vi "TreeItem.Property.Set.vi"(4 "Set String as Binary":bool, 8 "error in (no error)":errorcluster, 9 "Value":variant, 10 "Property Name":string, 11 "BaseNodeType":refnum<k24>) -> (0 "error out":errorcluster, 1 "Replaced":bool, 3 "BaseNodeType":refnum<k24>)   [LabVIEW 2015, in "Advanced System Definition.lvlib"]
doc: "Saves the new values/items into their corresponding position within the Custom Device Hierarchy according to their corresponding data type."
uses:
  SysDef API/Advanced System Definition.lvlib
  NationalInstruments.VeriStand.SystemStorage
  _Types/Property.DependentFile.ctl
  <vilib>/NI Veristand/Custom Device API/Custom Device Item Ref.ctl
  NationalInstruments.VeriStand.SystemDefinitionAPI
  <vilib>/Utility/VariantDataType/VariantType.lvlib
  <vilib>/NI Veristand/Custom Device API/Custom Device API.lvlib
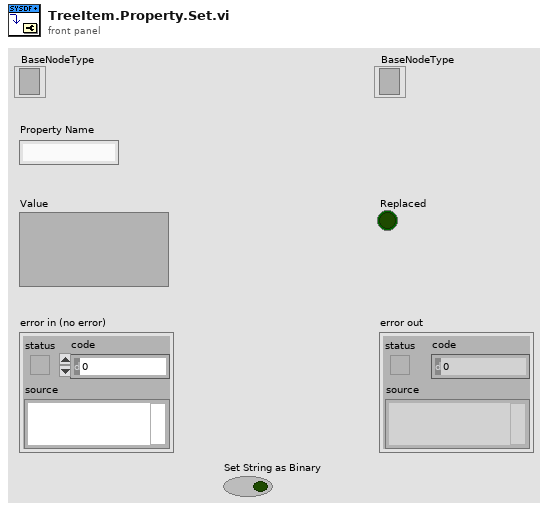
[diagram p1: front panel]
types:
  T1 = typedef "VariantType.lvlib/Type.ctl" = enum8{"Invalid Type", "Void", "I8", "I16", "I32", "I64", "U8", "U16", "U32", "U64", "Single Float", "Double Float", "Extended Float", "Single Complex", "Double Complex", "Extended Complex", "Enum U8", "Enum U16", "Enum U32", "Enum U64", "Single Float With Unit", "Double Float With Unit", "Extended Float With Unit", "Single Complex with Unit", "Double Complex with Unit", "Extended Complex with Unit", "Boolean", "String", "Path", "Picture", "Tag", "Array", "Cluster", "Variant", "LV Variant", "Waveform", "Timestamp", "Digital Waveform", "Digital Data", "ExpressData", "Refnum", "External Data", "VI", "Poly VI", "LabVIEW Class Instance", "Fixed Point"}
  T2 = typedef "Advanced System Definition.lvlib/Property.DependentFile.ctl" = cluster{"Original Path":path, "Version":string, "RTDestination":path, "ForceDownload":bool, "SupportedTarget":string, "MD5":string}
  T3 = typedef "Custom Device API.lvlib/Custom Device Item Ref.ctl" = u64
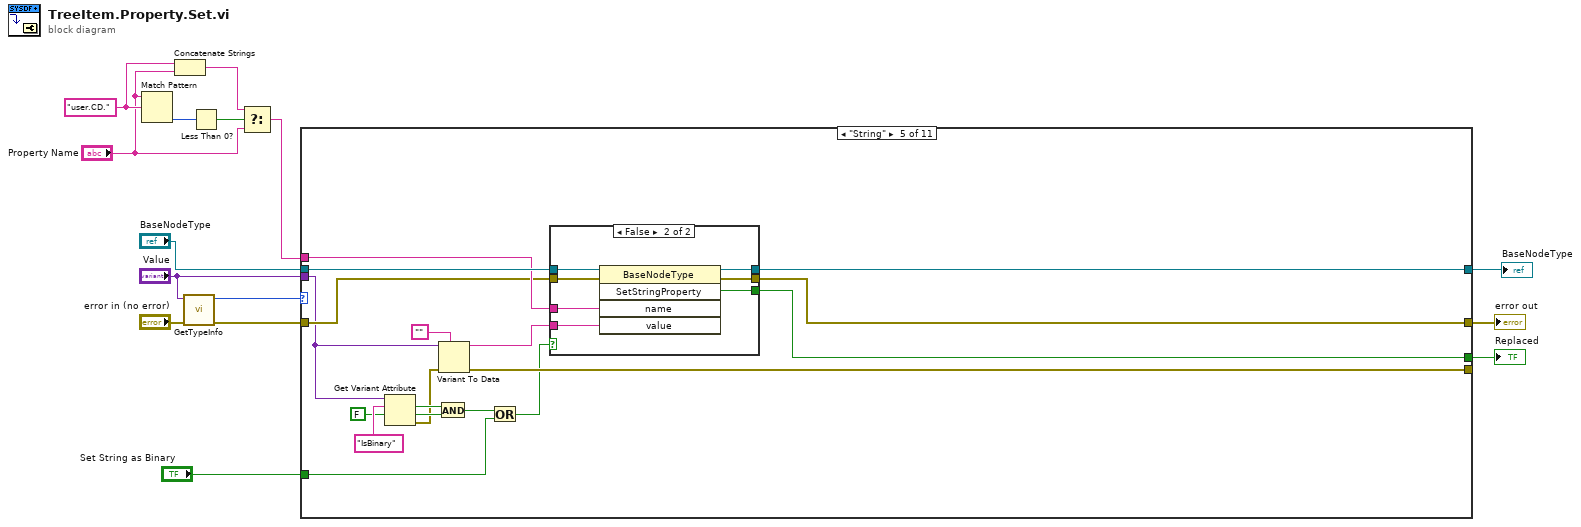
[diagram p0: block diagram]
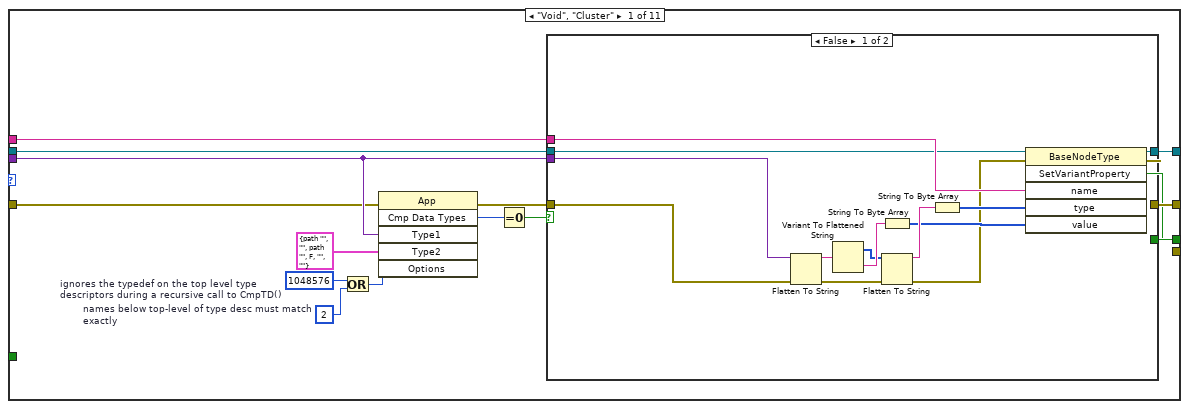
[diagram p2: hidden frame]
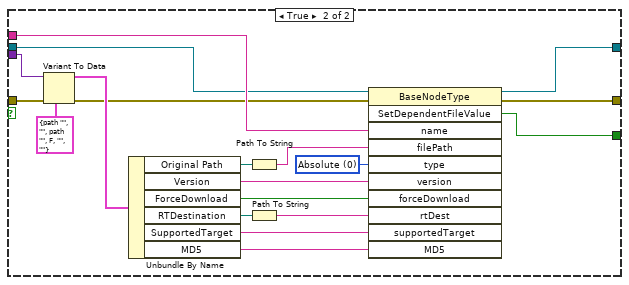
[diagram p3: hidden frame]
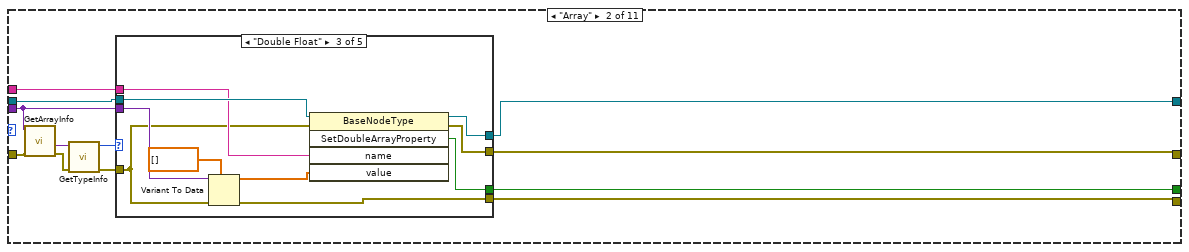
[diagram p4: hidden frame]
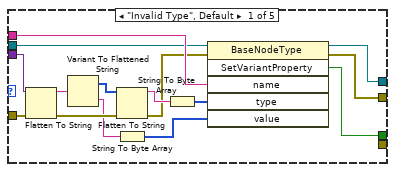
[diagram p5: hidden frame]
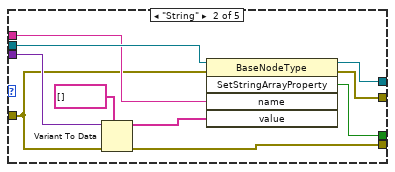
[diagram p6: hidden frame]
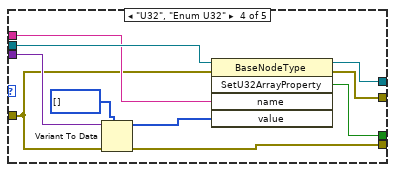
[diagram p7: hidden frame]
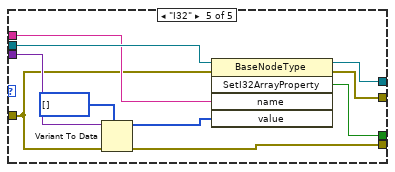
[diagram p8: hidden frame]
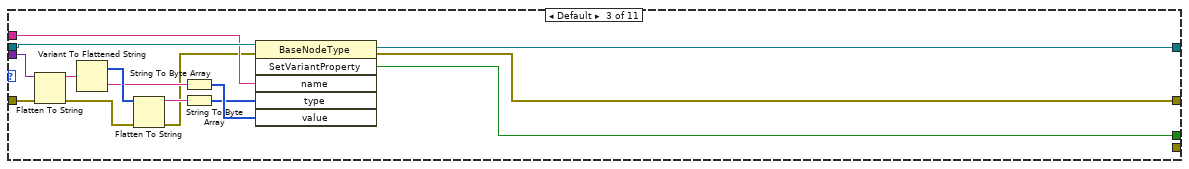
[diagram p9: hidden frame]
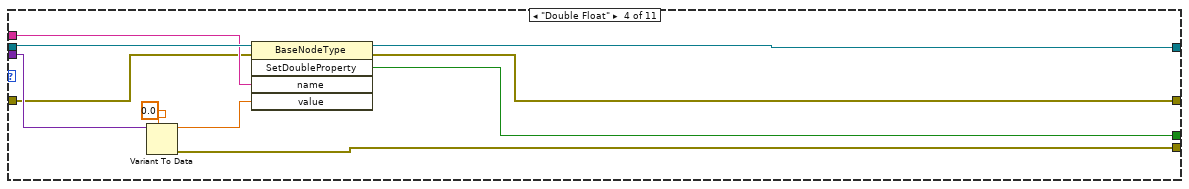
[diagram p10: hidden frame]
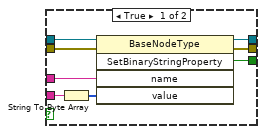
[diagram p11: hidden frame]
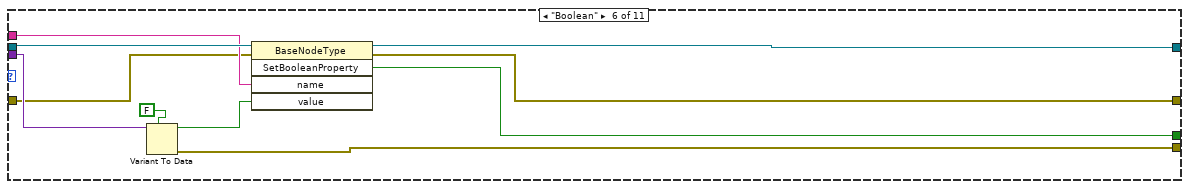
[diagram p12: hidden frame]
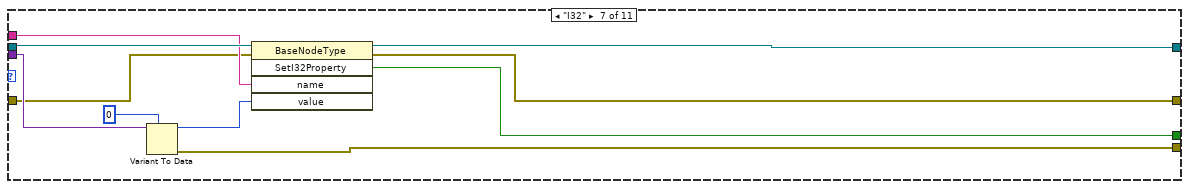
[diagram p13: hidden frame]
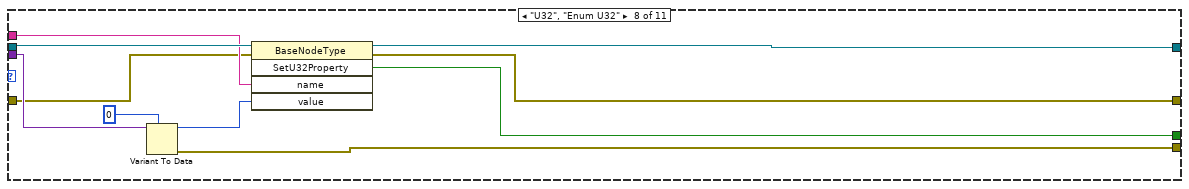
[diagram p14: hidden frame]
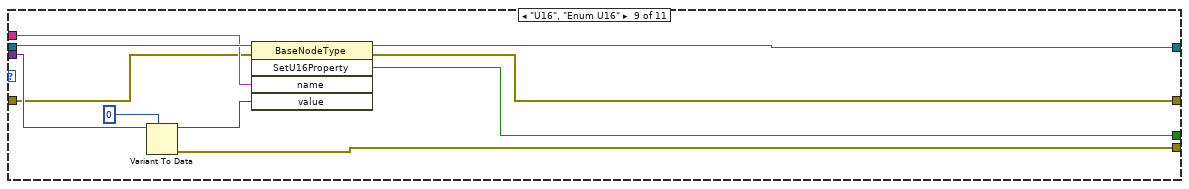
[diagram p15: hidden frame]
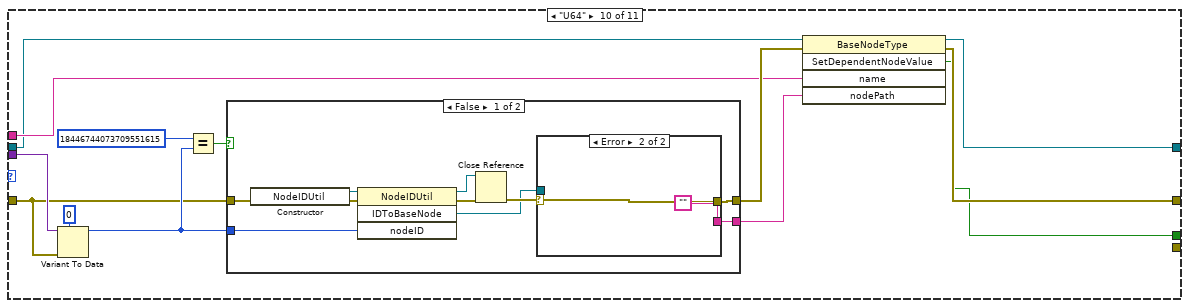
[diagram p16: hidden frame]
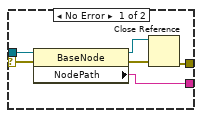
[diagram p17: hidden frame]
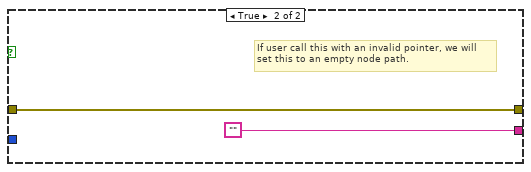
[diagram p18: hidden frame]
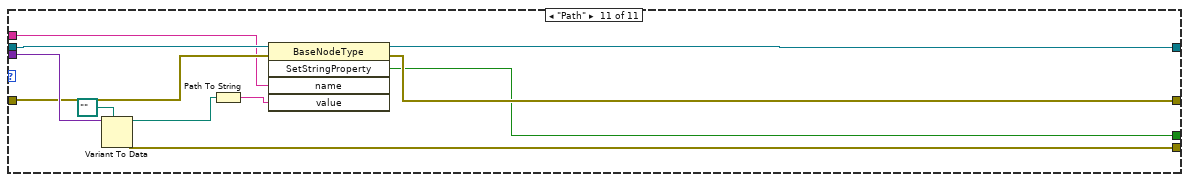
[diagram p19: hidden frame]
diagram:
  w3 = "user.CD." ("regular expression")
  n1 = Match Pattern(string="Property Name", regular expression=w3) -> (offset past match=w6:i32)  [unwired: 1 in, 3 out]
  n2 = Concatenate Strings(w3, "Property Name") -> (w4:string)
  n3 = call <vilib>:"GetTypeInfo.vi"("error in (no error)"="error in (no error)", "Variant"="Value") -> ("error out"=w11:errorcluster, "Type Enum"=w15:T1)  [unwired: 5 in, 3 out]
  n4 = Less Than 0?(x=w6) -> (x < 0?=w5:bool)
  n5 = Select(t=w4, s=w5, f="Property Name") -> (s? t:f=w1:string)
  n6 = case shown="\"String\"" w15 {
    tunnel: "BaseNodeType" -> [w28 w70 w145 w152 w172 w195 w205 w215 w225 w232 w269]
    tunnel: w11 -> [w17 w75 w135 w150 w170 w193 w203 w213 w223 w235 w268]
    tunnel: [w27 w68 w143 w149 w169 w192 w202 w212 w222 w231 w264] -> w14
    tunnel: w1 -> [w29 w69 w144 w151 w171 w194 w204 w214 w224 w233 w266]
    tunnel: "Value" -> [w20 w64 w134 w155 w157 w198 w208 w218 w228 w241 w272]
    tunnel: [w26 w67 w142 w148 w168 w191 w201 w211 w221 w229 w263] -> w13
    tunnel: [_ w66 _ w153 w173 w196 w206 w216 w226 _ w267] -> _
    tunnel: [w25 w65 w141 w146 w166 w189 w199 w209 w219 w230 w262] -> w8
    tunnel: "Set String as Binary" -> [_ _ _ _ w159 _ _ _ _ _ _]
    frame "Void", "Cluster" {
      w23 = 2  # names below top-level of type desc must match exactly
      w22 = 1048576  # ignores the typedef on the top level type descriptors during a recursive call to CmpTD()
      n7 = Or(x=w22, y=w23) -> (x .or. y?=w24:i32)
      n8 = invoke class="App" method="Cmp Data Types"(error in=w17, "Type1"=w20, "Type2"=T2 {"Original Path"=path "", "Version"="", "RTDestination"=path "", "ForceDownload"=FALSE, "SupportedTarget"="", "MD5"=""} ("OptionalInfo"), "Options"=w24) -> (error out=w16:errorcluster, "Compare Data Types"=w21:i32)  [unwired: 2 in, 4 out]
      n9 = Equal To 0?(x=w21) -> (x = 0?=w18:bool)
      n10 = case shown="False" w18 {
        tunnel: w29 -> [w44 w58]
        tunnel: w28 -> [w43 w56]
        tunnel: [w42 w47] -> w27
        tunnel: [w41 w46] -> w26
        tunnel: [w40 w55] -> w25
        tunnel: w16 -> [w34 w62]
        tunnel: w20 -> [w30 w63]
        frame False {
          n11 = Flatten To String(anything=w30, error in (no error)=w34) -> (data string=w36:string, error out=w35:errorcluster)  [unwired: 2 in, 1 out]
          n12 = Variant To Flattened String(Variant=w36) -> (data string=w39:string, 1:w37:i16[])
          n13 = String To Byte Array(string=w39) -> (unsigned byte array=w33:u8[])
          n14 = Flatten To String(anything=w37, error in (no error)=w35) -> (data string=w38:string, error out=w31:errorcluster)  [unwired: 2 in, 1 out]
          n15 = String To Byte Array(string=w38) -> (unsigned byte array=w32:u8[])
          n16 = invoke class="BaseNodeType" method="SetVariantProperty"(reference=w43, error in=w31, "name"=w44, "type"=w32, "value"=w33) -> (reference out=w40:refnum<k24>, error out=w42:errorcluster, "SetVariantProperty"=w41:bool)  [unwired: 1 in, 3 out]
        }
        frame True {
          w45 = 0 items=["Absolute", "Relative", "ToCommonDocDir", "ToApplicationDataDir"] ("type")
          n17 = Variant To Data(error in=w62, type=T2 {"Original Path"=path "", "Version"="", "RTDestination"=path "", "ForceDownload"=FALSE, "SupportedTarget"="", "MD5"=""} ("OptionalInfo"), Variant=w63) -> (data=w59:T2, error out=w48:errorcluster)
          n18 = Unbundle By Name(w59) -> ("Original Path"=w57:path, "Version"=w53:string, "ForceDownload"=w52:bool, "RTDestination"=w60:path, "SupportedTarget"=w50:string, "MD5"=w49:string)
          n19 = Path To String(path=w57) -> (string=w54:string)
          n20 = Path To String(path=w60) -> (string=w51:string)
          n21 = invoke class="BaseNodeType" method="SetDependentFileValue"(reference=w56, error in=w48, "name"=w58, "filePath"=w54, "type"=w45, "version"=w53, "forceDownload"=w52, "rtDest"=w51, "supportedTarget"=w50, "MD5"=w49) -> (reference out=w55:refnum<k24>, error out=w47:errorcluster, "SetDependentFileValue"=w46:bool)  [unwired: 1 in, 8 out]
        }
      }
    }
    frame "Array" {
      n22 = call <vilib>:"GetArrayInfo.vi"("error in (no error)"=w75, "Variant"=w64) -> ("error out"=w73:errorcluster, "ArrayElement"=w74:variant)  [unwired: 6 in, 2 out]
      n23 = call <vilib>:"GetTypeInfo.vi"("error in (no error)"=w73, "Variant"=w74) -> ("error out"=w71:errorcluster, "Type Enum"=w72:T1)  [unwired: 5 in, 3 out]
      n24 = case shown="\"Double Float\"" w72 {
        tunnel: w71 -> [w77 w93 w105 w114 w125]
        tunnel: w64 -> [w78 w100 w110 w120 w130]
        tunnel: w70 -> [w89 w97 w108 w118 w128]
        tunnel: w69 -> [w90 w95 w106 w116 w126]
        tunnel: [w88 w96 w107 w117 w127] -> w65
        tunnel: [w87 w91 w103 w112 w123] -> w68
        tunnel: [w86 w92 w104 w113 w124] -> w67
        tunnel: [_ w98 w109 w119 w129] -> w66
        frame "Invalid Type", Default {
          n25 = Flatten To String(anything=w78, error in (no error)=w77) -> (data string=w84:string, error out=w85:errorcluster)  [unwired: 2 in, 1 out]
          n26 = Variant To Flattened String(Variant=w84) -> (data string=w81:string, 1:w83:i16[])
          n27 = Flatten To String(anything=w83, error in (no error)=w85) -> (data string=w82:string, error out=w76:errorcluster)  [unwired: 2 in, 1 out]
          n28 = String To Byte Array(string=w81) -> (unsigned byte array=w79:u8[])
          n29 = String To Byte Array(string=w82) -> (unsigned byte array=w80:u8[])
          n30 = invoke class="BaseNodeType" method="SetVariantProperty"(reference=w89, error in=w76, "name"=w90, "type"=w80, "value"=w79) -> (reference out=w88:refnum<k24>, error out=w87:errorcluster, "SetVariantProperty"=w86:bool)  [unwired: 1 in, 3 out]
        }
        frame "String" {
          n31 = Variant To Data(error in=w93, type=string[] [], Variant=w100) -> (data=w94:string[], error out=w98:errorcluster)
          n32 = invoke class="BaseNodeType" method="SetStringArrayProperty"(reference=w97, error in=w93, "name"=w95, "value"=w94) -> (reference out=w96:refnum<k24>, error out=w91:errorcluster, "SetStringArrayProperty"=w92:bool)  [unwired: 1 in, 2 out]
        }
        frame "Double Float" {
          n33 = Variant To Data(error in=w105, type=dbl[] [], Variant=w110) -> (data=w101:dbl[], error out=w109:errorcluster)
          n34 = invoke class="BaseNodeType" method="SetDoubleArrayProperty"(reference=w108, error in=w105, "name"=w106, "value"=w101) -> (reference out=w107:refnum<k24>, error out=w103:errorcluster, "SetDoubleArrayProperty"=w104:bool)  [unwired: 1 in, 2 out]
        }
        frame "U32", "Enum U32" {
          n35 = Variant To Data(error in=w114, type=u32[] [], Variant=w120) -> (data=w115:u32[], error out=w119:errorcluster)
          n36 = invoke class="BaseNodeType" method="SetU32ArrayProperty"(reference=w118, error in=w114, "name"=w116, "value"=w115) -> (reference out=w117:refnum<k24>, error out=w112:errorcluster, "SetU32ArrayProperty"=w113:bool)  [unwired: 1 in, 2 out]
        }
        frame "I32" {
          n37 = Variant To Data(error in=w125, type=i32[] [], Variant=w130) -> (data=w121:i32[], error out=w129:errorcluster)
          n38 = invoke class="BaseNodeType" method="SetI32ArrayProperty"(reference=w128, error in=w125, "name"=w126, "value"=w121) -> (reference out=w127:refnum<k24>, error out=w123:errorcluster, "SetI32ArrayProperty"=w124:bool)  [unwired: 1 in, 2 out]
        }
      }
    }
    frame Default {
      n39 = Flatten To String(anything=w134, error in (no error)=w135) -> (data string=w139:string, error out=w140:errorcluster)  [unwired: 2 in, 1 out]
      n40 = Variant To Flattened String(Variant=w139) -> (data string=w136:string, 1:w138:i16[])
      n41 = Flatten To String(anything=w138, error in (no error)=w140) -> (data string=w137:string, error out=w133:errorcluster)  [unwired: 2 in, 1 out]
      n42 = String To Byte Array(string=w136) -> (unsigned byte array=w132:u8[])
      n43 = String To Byte Array(string=w137) -> (unsigned byte array=w131:u8[])
      n44 = invoke class="BaseNodeType" method="SetVariantProperty"(reference=w145, error in=w133, "name"=w144, "type"=w131, "value"=w132) -> (reference out=w141:refnum<k24>, error out=w143:errorcluster, "SetVariantProperty"=w142:bool)  [unwired: 1 in, 3 out]
    }
    frame "Double Float" {
      n45 = Variant To Data(type=0.0, Variant=w155) -> (data=w147:dbl, error out=w153:errorcluster)  [unwired: 1 in]
      n46 = invoke class="BaseNodeType" method="SetDoubleProperty"(reference=w152, error in=w150, "name"=w151, "value"=w147) -> (reference out=w146:refnum<k24>, error out=w149:errorcluster, "SetDoubleProperty"=w148:bool)  [unwired: 1 in, 2 out]
    }
    frame "String" {
      n47 = Get Variant Attribute(Variant=w157, name="IsBinary", default value (empty Variant)=FALSE ("Set String as Binary")) -> (found=w162:bool, value=w163:bool, error out=w156:errorcluster)  [unwired: 1 in, 1 out]
      n48 = And(x=w162, y=w163) -> (x .and. y?=w164:bool)
      n49 = Variant To Data(error in=w156, type="", Variant=w157) -> (data=w167:string, error out=w173:errorcluster)
      n50 = Or(x=w164, y=w159) -> (x .or. y?=w158:bool)
      n51 = case shown="False" w158 {
        tunnel: w172 -> [w181 w188]
        tunnel: w171 -> [w180 w187]
        tunnel: w170 -> [w179 w186]
        tunnel: [w178 w185] -> w169
        tunnel: [w177 w184] -> w168
        tunnel: w167 -> [w176 w183]
        tunnel: [w175 w182] -> w166
        frame True {
          n52 = String To Byte Array(string=w176) -> (unsigned byte array=w174:u8[])
          n53 = invoke class="BaseNodeType" method="SetBinaryStringProperty"(reference=w181, error in=w179, "name"=w180, "value"=w174) -> (reference out=w175:refnum<k24>, error out=w178:errorcluster, "SetBinaryStringProperty"=w177:bool)  [unwired: 1 in, 2 out]
        }
        frame False {
          n54 = invoke class="BaseNodeType" method="SetStringProperty"(reference=w188, error in=w186, "name"=w187, "value"=w183) -> (reference out=w182:refnum<k24>, error out=w185:errorcluster, "SetStringProperty"=w184:bool)  [unwired: 1 in, 2 out]
        }
      }
    }
    frame "Boolean" {
      n55 = Variant To Data(type=FALSE, Variant=w198) -> (data=w190:bool, error out=w196:errorcluster)  [unwired: 1 in]
      n56 = invoke class="BaseNodeType" method="SetBooleanProperty"(reference=w195, error in=w193, "name"=w194, "value"=w190) -> (reference out=w189:refnum<k24>, error out=w192:errorcluster, "SetBooleanProperty"=w191:bool)  [unwired: 1 in, 2 out]
    }
    frame "I32" {
      n57 = Variant To Data(type=0, Variant=w208) -> (data=w200:i32, error out=w206:errorcluster)  [unwired: 1 in]
      n58 = invoke class="BaseNodeType" method="SetI32Property"(reference=w205, error in=w203, "name"=w204, "value"=w200) -> (reference out=w199:refnum<k24>, error out=w202:errorcluster, "SetI32Property"=w201:bool)  [unwired: 1 in, 2 out]
    }
    frame "U32", "Enum U32" {
      n59 = Variant To Data(type=u32 0, Variant=w218) -> (data=w210:u32, error out=w216:errorcluster)  [unwired: 1 in]
      n60 = invoke class="BaseNodeType" method="SetU32Property"(reference=w215, error in=w213, "name"=w214, "value"=w210) -> (reference out=w209:refnum<k24>, error out=w212:errorcluster, "SetU32Property"=w211:bool)  [unwired: 1 in, 2 out]
    }
    frame "U16", "Enum U16" {
      n61 = Variant To Data(type=u16 0, Variant=w228) -> (data=w220:u16, error out=w226:errorcluster)  [unwired: 1 in]
      n62 = invoke class="BaseNodeType" method="SetU16Property"(reference=w225, error in=w223, "name"=w224, "value"=w220) -> (reference out=w219:refnum<k24>, error out=w222:errorcluster, "SetU16Property"=w221:bool)  [unwired: 1 in, 2 out]
    }
    frame "U64" {
      n63 = Variant To Data(error in=w235, type=u64 0, Variant=w241) -> (data=w236:u64)  [unwired: 1 out]
      n64 = Equal?(x=T3 18446744073709551615 ("Dependent Node Ref"), y=w236) -> (x = y?=w238:bool)
      n65 = case shown="False" w238 {
        tunnel: [w251 ""] -> w237
        tunnel: w236 -> [w244 _]
        tunnel: w235 -> [w243 w260]
        tunnel: [w242 w260] -> w234
        frame False {
          n66 = constructor class="NodeIDUtil"(error in=w243) -> (reference out=w247:refnum<k24>, error out=w248:errorcluster)  [unwired: 2 in, 1 out]
          n67 = invoke class="NodeIDUtil" method="IDToBaseNode"(reference=w247, error in=w248, "nodeID"=w244) -> (reference out=w250:refnum<k24>, error out=w249:errorcluster, "IDToBaseNode"=w245:refnum<k24>)  [unwired: 1 in, 1 out]
          n68 = Close Reference(reference=w250, error in (no error)=w249) -> (error out=w246:errorcluster)
          n69 = case shown="Error" w246 {
            selector: w246 -> [w253 w258]
            tunnel: w245 -> [w257 _]
            tunnel: [w256 ""] -> w251
            tunnel: [w252 w258] -> w242
            frame No Error {
              n70 = property class="BaseNode"(reference=w257, error in=w253) -> (reference out=w254:refnum<k24>, error out=w255:errorcluster, "NodePath"=w256:string)
              n71 = Close Reference(reference=w254, error in (no error)=w255) -> (error out=w252:errorcluster)
            }
            frame Error {
            }
          }
        }
        frame True {
          # "If user call this with an invalid pointer, we will\nset this to an empty node path."
        }
      }
      n72 = invoke class="BaseNodeType" method="SetDependentNodeValue"(reference=w232, error in=w234, "name"=w233, "nodePath"=w237) -> (reference out=w230:refnum<k24>, error out=w231:errorcluster, "SetDependentNodeValue"=w229:bool)  [unwired: 1 in, 2 out]
    }
    frame "Path" {
      n73 = Variant To Data(type=path "", Variant=w272) -> (data=w270:path, error out=w267:errorcluster)  [unwired: 1 in]
      n74 = Path To String(path=w270) -> (string=w265:string)
      n75 = invoke class="BaseNodeType" method="SetStringProperty"(reference=w269, error in=w268, "name"=w266, "value"=w265) -> (reference out=w262:refnum<k24>, error out=w264:errorcluster, "SetStringProperty"=w263:bool)  [unwired: 1 in, 2 out]
    }
  }
  "Replaced" <- w13
  "error out" <- w14
  "BaseNodeType" <- w8
